vi "Read AVI to Array.vi"(0 "AVI Path":path, 1 "Error in (no error)":errorcluster) -> (2 "Image Array":T1[](array[plugin-control]), 3 "Data Array":string[](array[string]), 4 "Error out":errorcluster)   [LabVIEW 2012]
doc: "This example shows how to read and write both image information and data to an AVI file. The example also shows how to read a specific frame in an AVI file. The VI opens an existing AVI file, adds time stamp information, sample waveform data, and writes a sample image and the data to a new AVI file. You then can read the image and data associated with a specific frame. Use the Flatten To String and Unflatten From String functions to write and read data in AVI files."
uses:
  <vilib>/vision/Image Controls.llb/IMAQ Image.ctl
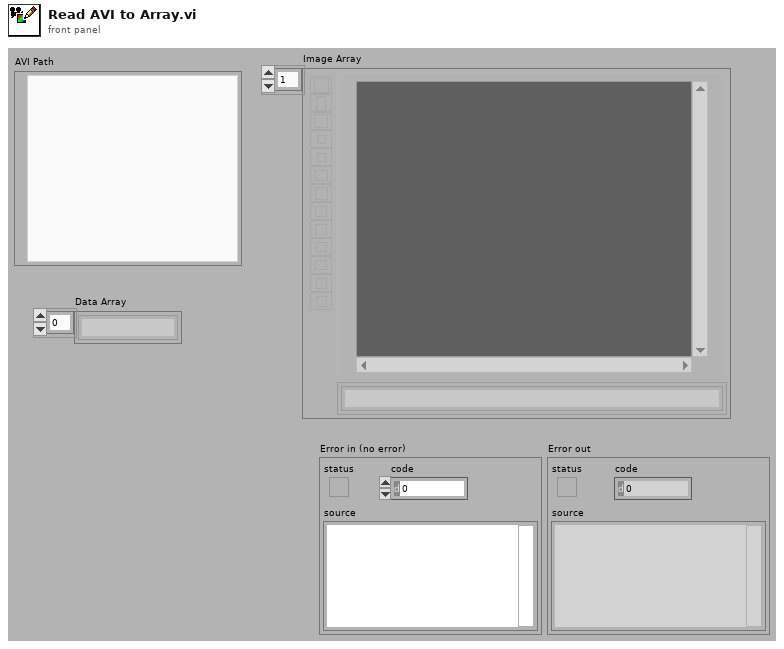
[diagram p1: front panel]
types:
  T1 = typedef "IMAQ Image.ctl" = refnum<image>
  T2 = typedef "Image Type" = u32
  T3 = typedef "AviRefnum.ctl" = refnum<k1>
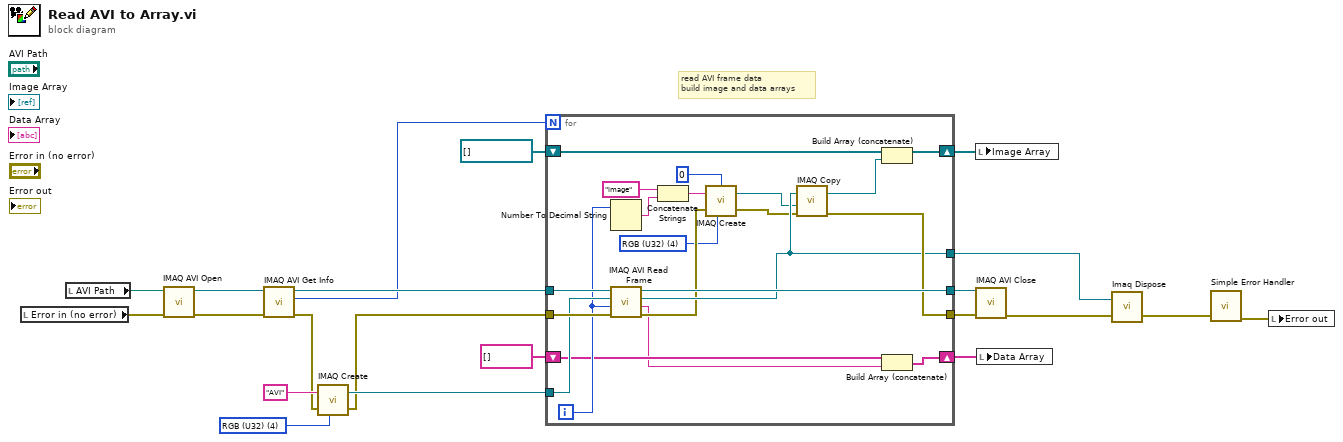
[diagram p0: block diagram]
diagram:
  w7 = T2 4 items=["Grayscale (U8)", "Grayscale (I16)", "Grayscale (SGL)", "Complex (CSG)", "RGB (U32)", "HSL (U32)", "RGB (U64)", "Grayscale (U16)"] ("Image Type")
  # "read AVI frame data\nbuild image and data arrays"
  n1 = local read "Error in (no error)"() -> (w21:errorcluster)
  n2 = local read "AVI Path"() -> (w8:path)
  n3 = call "IMAQ AVI Open"("error in (no error)"=w21, "AVI Path"=w8) -> ("error out"=w12:errorcluster, "Avi Refnum"=w11:T3)  [unwired: 8 out]
  n4 = call "IMAQ AVI Get Info"("error in (no error)"=w12, "Avi Refnum"=w11) -> ("error out"=w5:errorcluster, "Number of Frames"=w6:u32, "Avi Refnum (duplicate)"=w10:T3)  [unwired: 5 in, 2 out]
  n5 = call "IMAQ Create"("Image Name"="AVI", "Image Type"=w7, "error in (no error)"=w5) -> ("New Image"=w17:T1, "error out"=w1:errorcluster)  [unwired: 1 in, 1 out]
  n6 = for {
    N: w6 -> [_]
    tunnel: [w37] -> w15
    tunnel: w17 -> [w38]
    tunnel: [w39] -> w14
    tunnel: [w40] -> w16
    tunnel: w10 -> [w42]
    tunnel: w1 -> [w41]
    shift-right: [w35] -> w3
    shift-left: T1[] [] ("Image Array") -> [w36]
    shift-right: [w24] -> w2
    shift-left: string[] [] ("Data Array") -> [w25]
    i -> [w26]
    w27 = T2 4 items=["Grayscale (U8)", "Grayscale (I16)", "Grayscale (SGL)", "Complex (CSG)", "RGB (U32)", "HSL (U32)", "RGB (U64)", "Grayscale (U16)"] ("Image Type")
    n7 = Number To Decimal String(number=w26) -> (decimal integer string=w32:string)  [unwired: 1 in]
    n8 = call "IMAQ AVI Read Frame"("error in (no error)"=w41, "Frame Number"=w26, "Image"=w38, "Avi Refnum"=w42) -> ("error out"=w29:errorcluster, "Data Out"=w22:string, "Image Out"=w37:T1, "Avi Refnum (duplicate)"=w40:T3)  [unwired: 1 in, 3 out]
    n9 = Concatenate Strings("image" ("string"), w32) -> (w34:string)
    n10 = call "IMAQ Create"("Border Size"=0, "Image Name"=w34, "Image Type"=w27, "error in (no error)"=w29) -> ("New Image"=w30:T1, "error out"=w28:errorcluster)  [unwired: 1 in]
    n11 = call "IMAQ Copy"("error in (no error)"=w28, "Image Dst"=w30, "Image Src"=w37) -> ("error out"=w39:errorcluster, "Image Dst Out"=w23:T1)  [unwired: 3 in]
    n12 = Build Array (concatenate)(w36, w23) -> (w35:T1[])
    n13 = Build Array (concatenate)(w25, w22) -> (w24:string[])
  }
  n14 = local write "Image Array"(w3) -> ()
  n15 = call "IMAQ AVI Close"("error in (no error)"=w14, "Avi Refnum"=w16) -> ("error out"=w13:errorcluster)  [unwired: 9 out]
  n16 = local write "Data Array"(w2) -> ()
  n17 = call "Imaq Dispose"("Image"=w15, "error in (no error)"=w13) -> ("error out"=w19:errorcluster)  [unwired: 1 in, 3 out]
  n18 = call <vilib>:"Simple Error Handler.vi"("error in (no error)"=w19) -> ("error out"=w20:errorcluster)  [unwired: 1 in, 7 out]
  n19 = local write "Error out"(w20) -> ()
